vi "Scripting_UpdateViFromTemplate.vi"(0 "ViRef":refnum<vi>, 1 "TemplateVI(Path or Ref)":variant, 5 "error in (no error)":errorcluster) -> (15 "TemplateVersionUsed":string, 19 "error out":errorcluster={"status"=TRUE, "code"=1055, "source"="Property Node in Scripting_ConvertBaseClassToSubClass.vi"})   [LabVIEW 2020]
uses:
  <vilib>/Utility/miscctls.llb/LVRectTypeDef.ctl
  <vilib>/Utility/miscctls.llb/LVPositionTypeDef.ctl
  b5d46679-8400-4ee0-8a03-e36cc4015ed4.vi
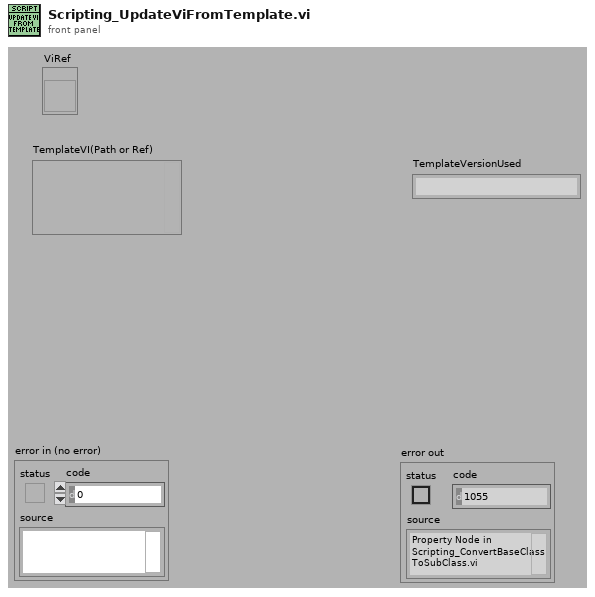
[diagram p1: front panel]
types:
  T1 = typedef "LVRectTypeDef.ctl" = cluster{"Left":i16, "Top":i16, "Right":i16, "Bottom":i16}
  T2 = typedef "LVPositionTypeDef.ctl" = cluster{"Left":i32, "Top":i32}
  T3 = cluster{"ViRef":refnum<vi>, "TemplateRef":refnum<vi>, "ConnectorPaneSettings":cluster{i32, "Wire Rule":enum16{"Invalid Wire Rule", "Required", "Recommended", "Optional", "Dynamic Dispatch"}}[], "ConnectorPaneControlsLabels":string[], "ViClassPath":path, "TemplateViClassPath":path, "ViRootBaseClassPath":path, "TemplateRootBaseClassPath":path, "ClassName":string, "TemplateMemberDataPath":path, "TemplateFile":path, "TemplateVersionUsed":string, "Class":refnum<vi>, "TemplateClassName":string, "permissions":i16, "TemplateClass":refnum<vi>, "Master Bounds Rect":T1, "Visible":bool[], "Controls":refnum<vi>[], "Positions":T2[]}
  T4 = enum32{"invalid lock state", "Not Locked", "Locked (No Password)", "Password-protected"}
  T5 = enum32{"invalid VI type", "Standard VI", "Control VI", "Global VI", "Polymorphic VI", "Configuration VI", "SubSystem", "Facade VI", "Method VI", "Statechart Diagram VI"}
  T6 = enum32{"invalid VI type", "Standard VI", "Control VI", "Global VI", "Polymorphic VI", "Configuration VI", "SubSystem", "Facade VI", "Method VI"}
  T7 = cluster{"Major":u16, "Minor":u16, "Fix":u16, "Build":u16}
  T8 = enum16{"Invalid Wire Rule", "Required", "Recommended", "Optional", "Dynamic Dispatch"}[]
  T9 = cluster{i32, "Wire Rule":enum16{"Invalid Wire Rule", "Required", "Recommended", "Optional", "Dynamic Dispatch"}}
  T10 = cluster{"Position":T2, "Label.Text":string, "Visible":bool, cluster{i32, "Wire Rule":enum16{"Invalid Wire Rule", "Required", "Recommended", "Optional", "Dynamic Dispatch"}}}
  T11 = cluster{"Position":T2, "Label.Text":string, "Visible":bool, cluster{i32, "Wire Rule":enum16{"Invalid Wire Rule", "Required", "Recommended", "Optional", "Dynamic Dispatch"}}}[]
  T12 = cluster{i32, "Wire Rule":enum16{"Invalid Wire Rule", "Required", "Recommended", "Optional", "Dynamic Dispatch"}}[]
  T13 = cluster{"Position":T2, refnum<vi>, "Label.Text":string}
  T14 = cluster{"Position":T2, refnum<vi>, "Label.Text":string}[]
  T15 = enum16{"Invalid Wire Rule", "Required", "Recommended", "Optional", "Dynamic Dispatch"}
  T16 = enum32{"Bad", "Idle", "Run top level", "Running"}
  T17 = typedef "LVPointTypeDef.ctl" = cluster{"Horizontal":i16, "Vertical":i16}
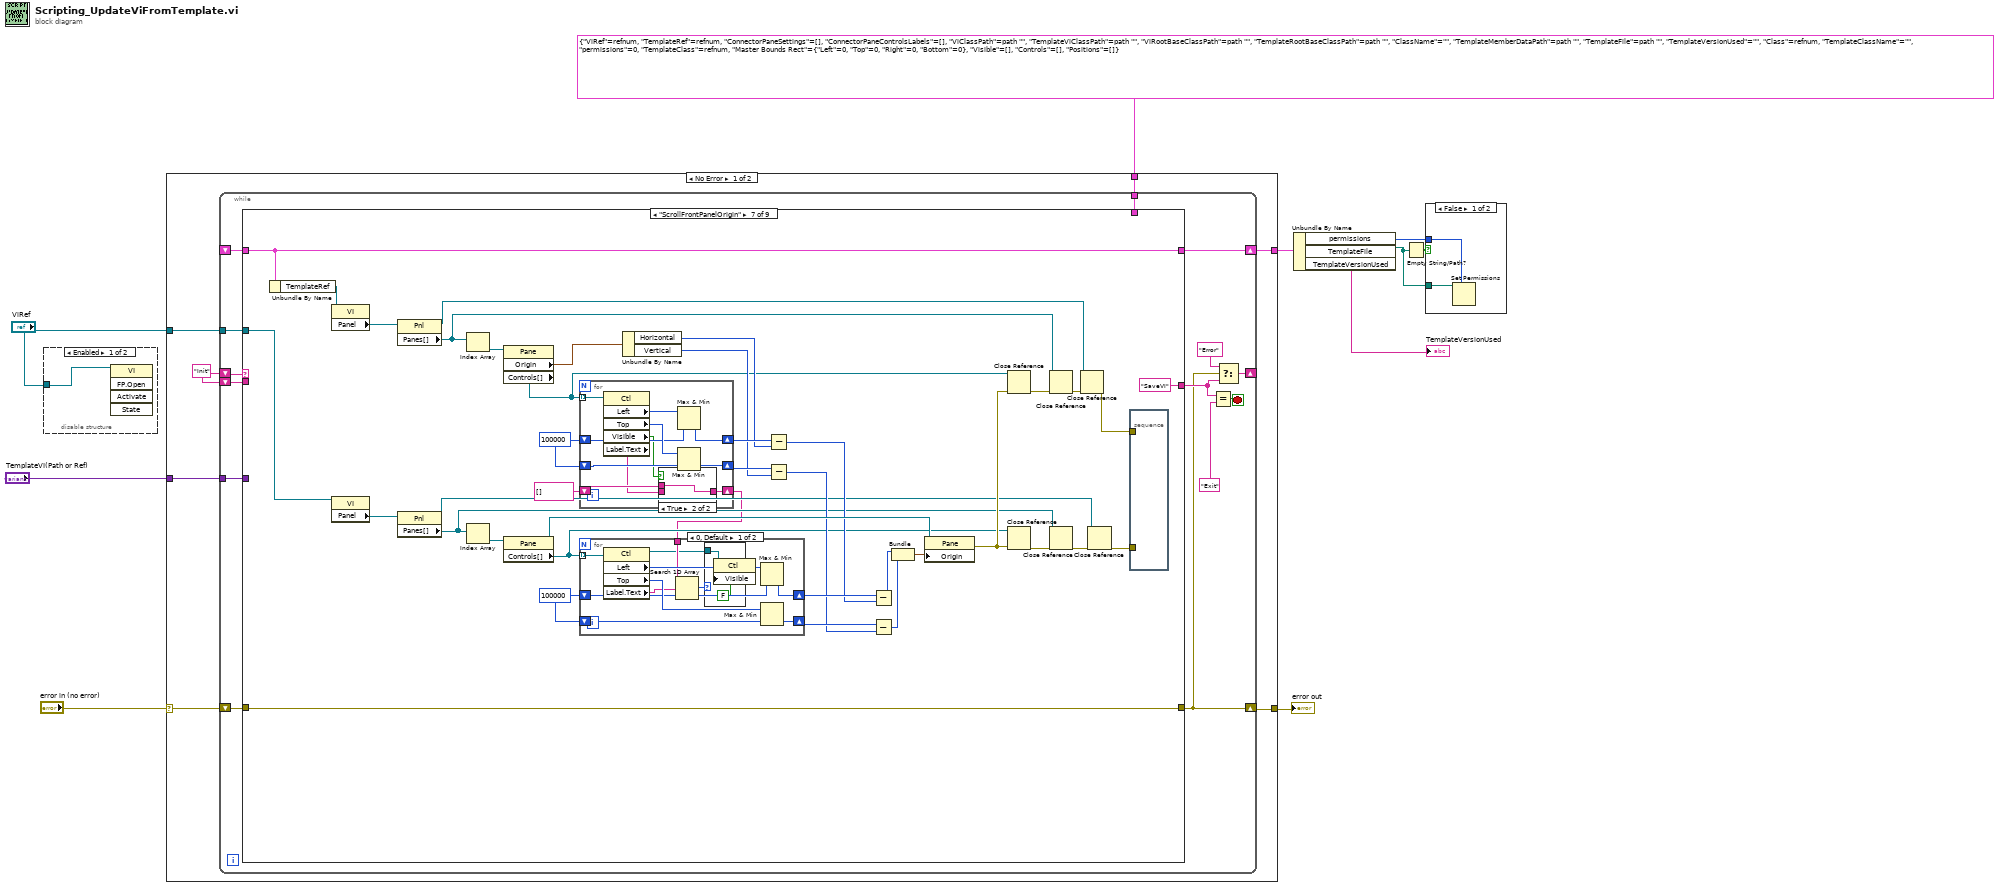
[diagram p0: block diagram]
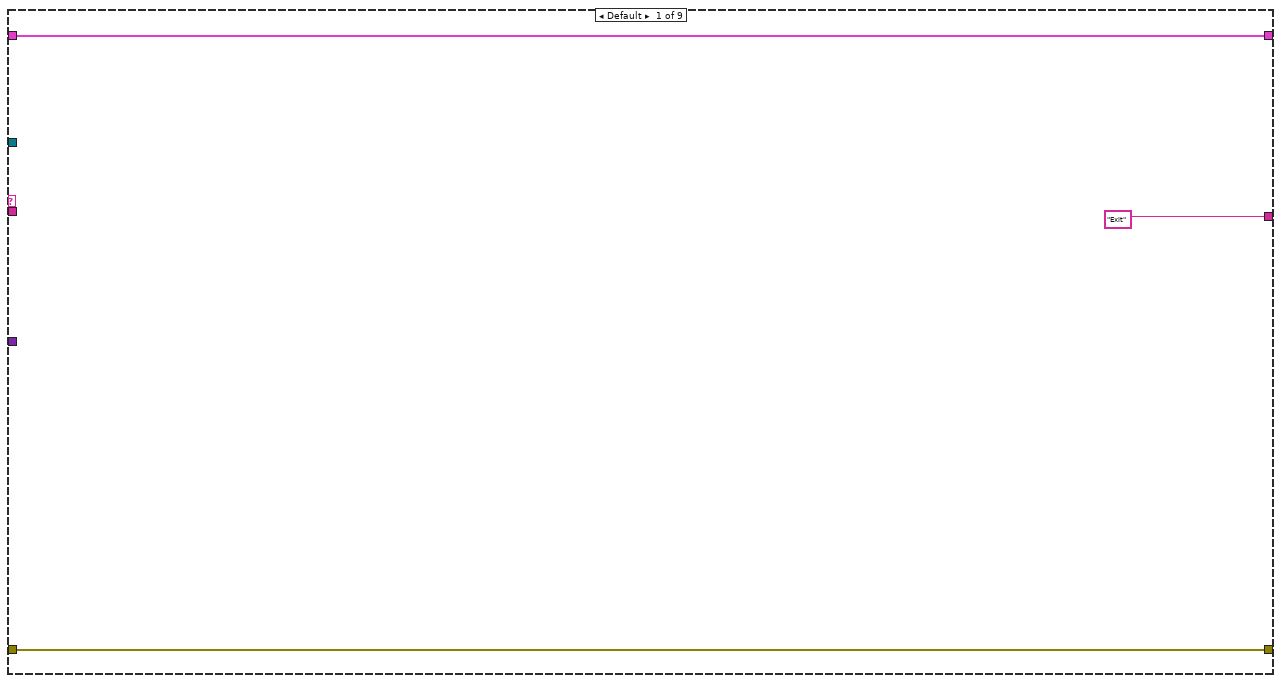
[diagram p4: hidden frame]
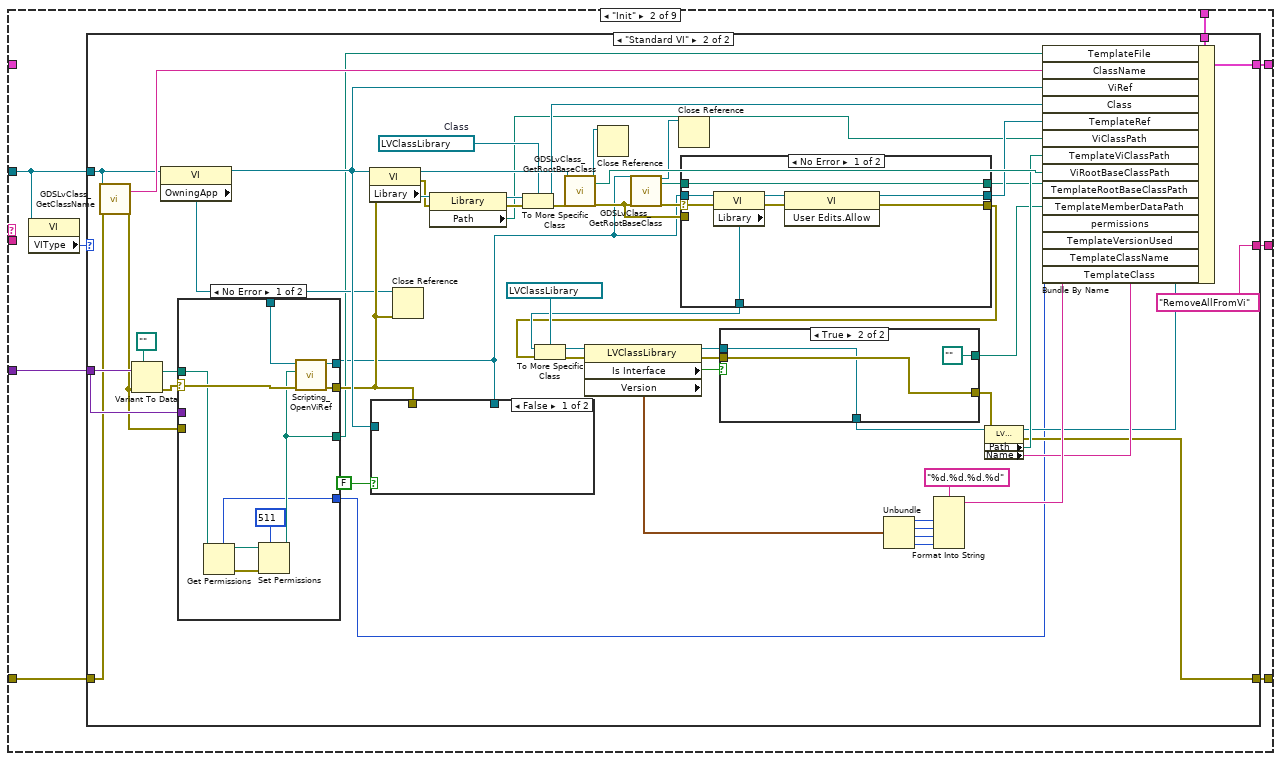
[diagram p5: hidden frame]
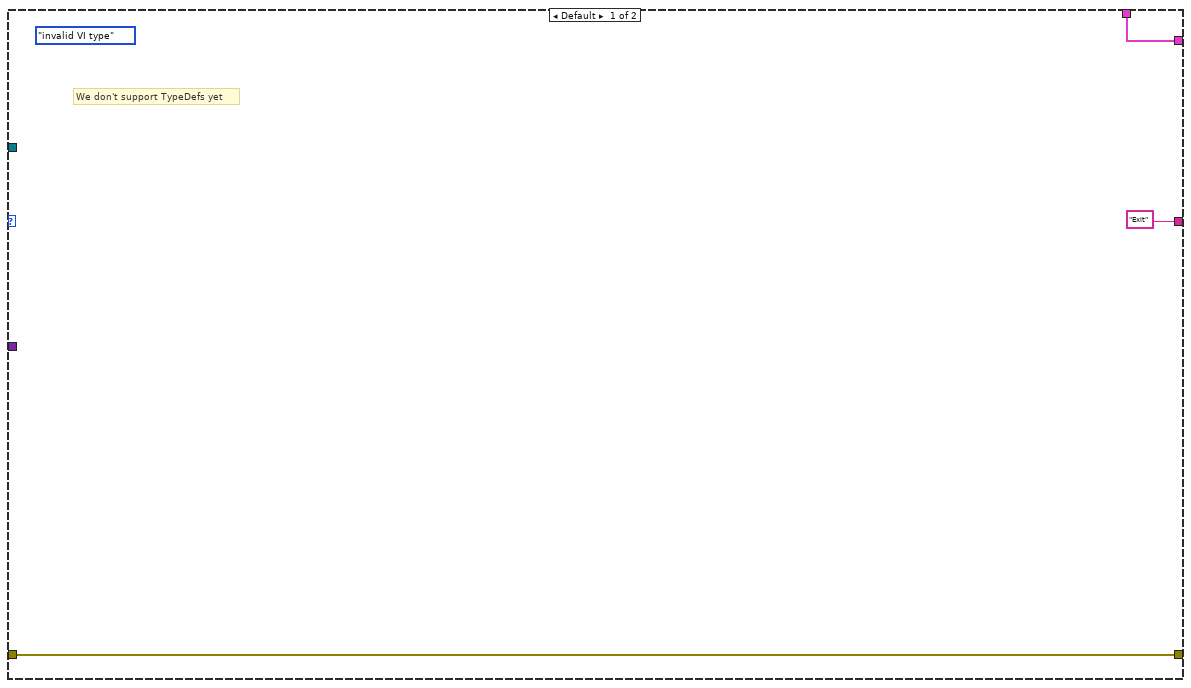
[diagram p6: hidden frame]
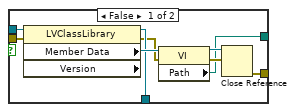
[diagram p7: hidden frame]
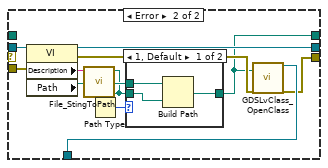
[diagram p8: hidden frame]
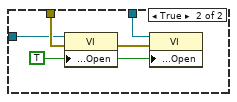
[diagram p10: hidden frame]
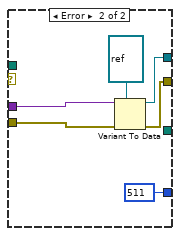
[diagram p11: hidden frame]
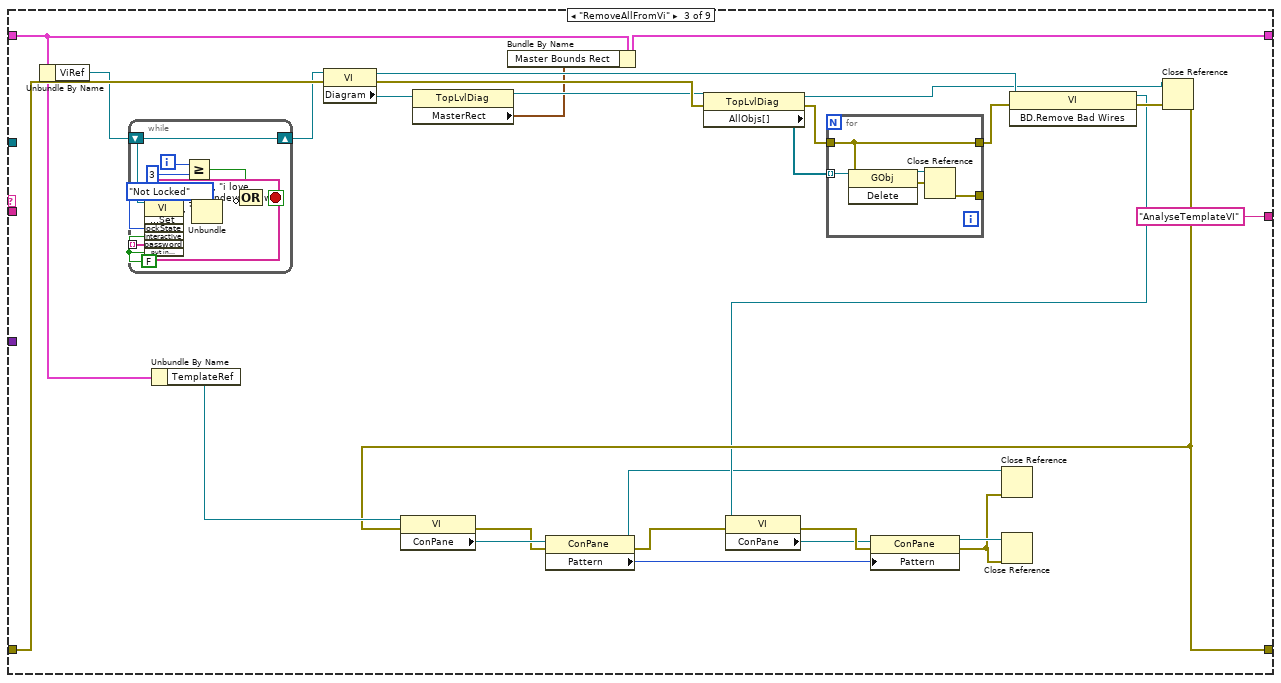
[diagram p12: hidden frame]
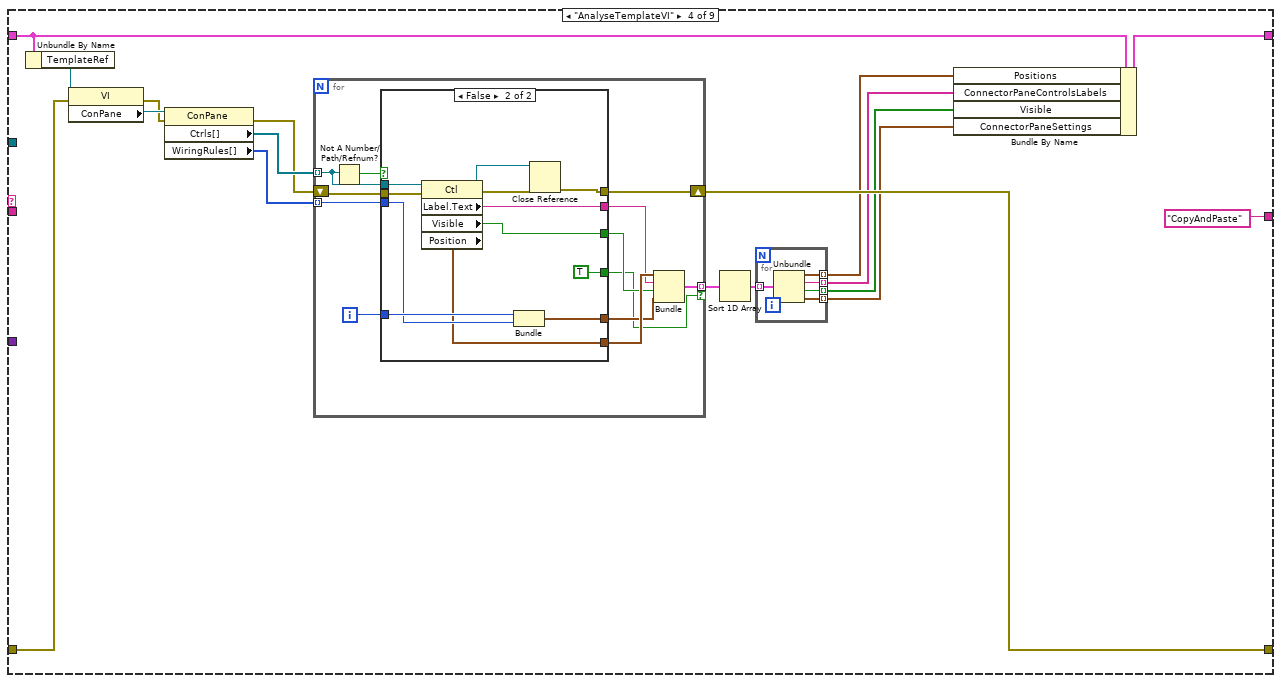
[diagram p13: hidden frame]
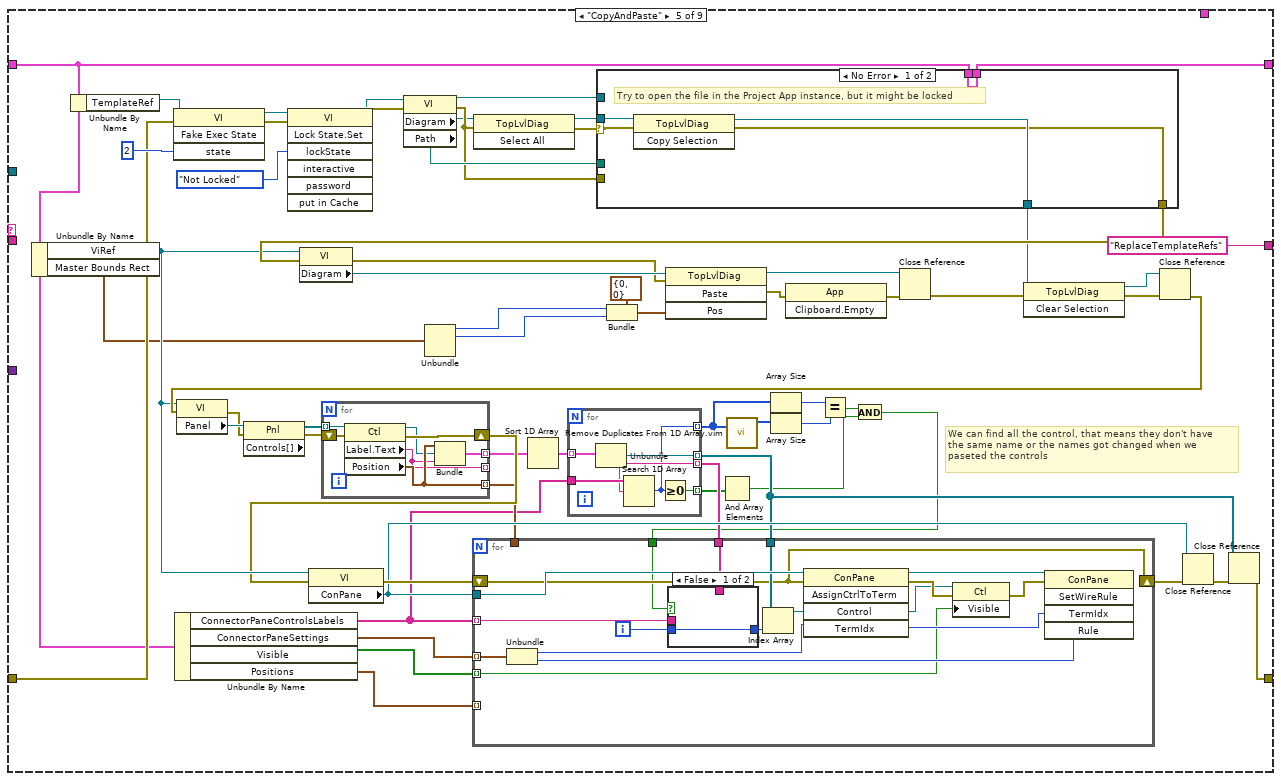
[diagram p15: hidden frame]
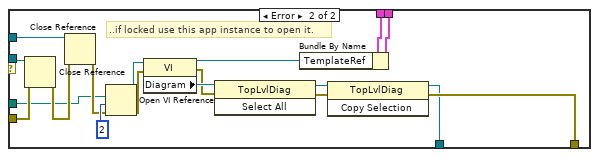
[diagram p16: hidden frame]
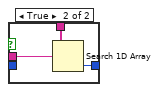
[diagram p17: hidden frame]
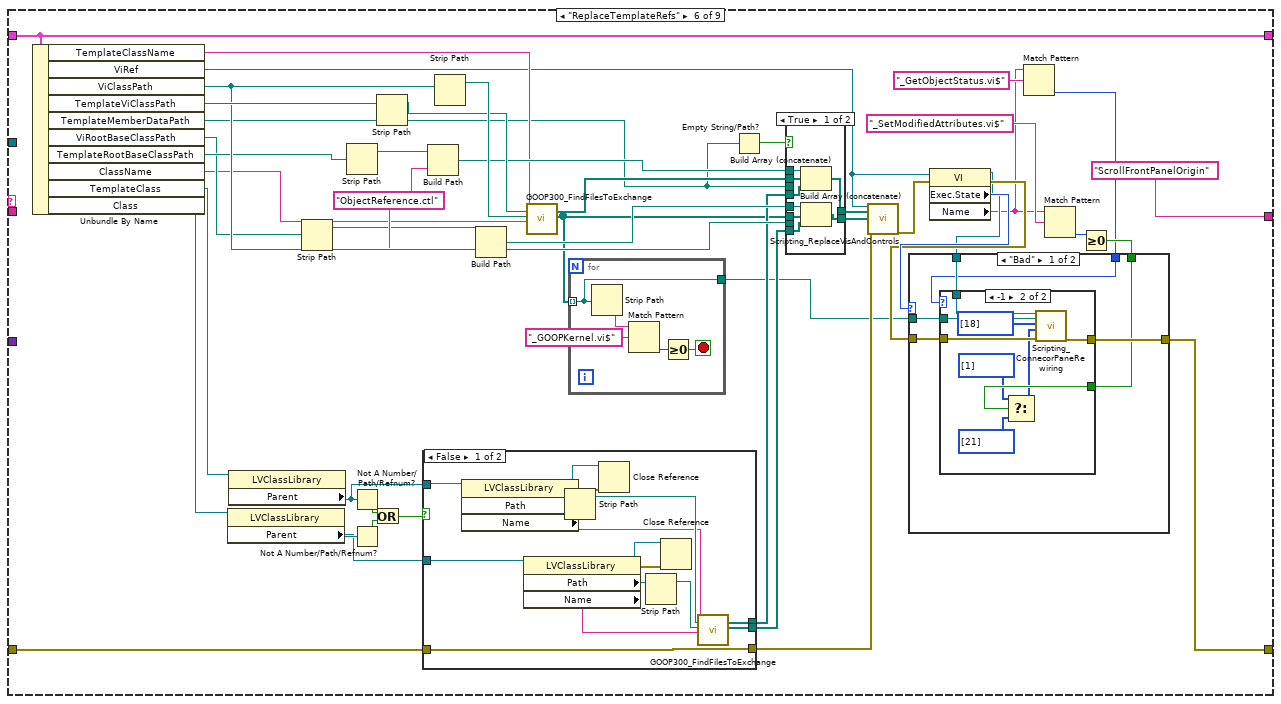
[diagram p18: hidden frame]
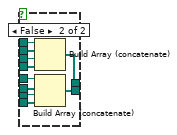
[diagram p19: hidden frame]
diagram:
  n1 = disable-structure shown="Enabled" {
    disable-tunnel: "ViRef" -> [w11 _]
    frame Enabled {
      n2 = invoke class="VI" method="FP.Open"(reference=w11) -> ()  [unwired: 4 in, 5 out]
    }
    frame Disabled {
    }
  }
  n3 = case shown="No Error" "error in (no error)" {
    selector: "error in (no error)" -> [w13 w583]
    tunnel: [w18 w583] -> w10
    tunnel: T3 {"ViRef"=refnum, "TemplateRef"=refnum, "ConnectorPaneSettings"=[], "ConnectorPaneControlsLabels"=[], "ViClassPath"=path "", "TemplateViClassPath"=path "", "ViRootBaseClassPath"=path "", "TemplateRootBaseClassPath"=path "", "ClassName"="", "TemplateMemberDataPath"=path "", "TemplateFile"=path "", "TemplateVersionUsed"="", "Class"=refnum, "TemplateClassName"="", "permissions"=0, "TemplateClass"=refnum, "Master Bounds Rect"={"Left"=0, "Top"=0, "Right"=0, "Bottom"=0}, "Visible"=[], "Controls"=[], "Positions"=[]} -> [w17 _]
    tunnel: "ViRef" -> [w16 _]
    tunnel: "TemplateVI(Path or Ref)" -> [w15 _]
    tunnel: [w12 _] -> w6
    frame No Error {
      w14 = "Init"
      n4 = while {
        shift-right: [w20] -> w18
        shift-left: w13 -> [w22]
        shift-right: [w32] -> _
        shift-left: w14 -> [w27]
        shift-right: [w21] -> w12
        shift-left: _ -> [w26]
        tunnel: w16 -> [w24]
        tunnel: w17 -> [w25]
        tunnel: w15 -> [w23]
        shift-left: w14 -> [w19]
        stop <- w31 stop-if-true
        n5 = case shown="\"ScrollFrontPanelOrigin\"" w27 {
          tunnel: w22 -> [w35 w39 w186 w215 w298 w374 w507 w538 w544]
          tunnel: [w35 w38 w167 w210 w268 w371 w507 w537 w547] -> w20
          tunnel: ["Exit" w43 "AnalyseTemplateVI" "CopyAndPaste" "ReplaceTemplateRefs" "ScrollFrontPanelOrigin" "SaveVI" "CloseReferences" "Exit"] -> w28
          tunnel: [w33 w42 w173 w217 w290 w373 w476 w540 w543] -> w21
          tunnel: w26 -> [w33 _ w171 w218 w284 w373 w476 w540 w543]
          tunnel: w24 -> [_ w37 _ _ _ _ w472 _ w552]
          tunnel: w25 -> [_ w41 _ _ _ _ _ _ _]
          tunnel: w23 -> [_ w40 _ _ _ _ _ _ w554]
          tunnel: w19 -> [_ _ _ _ _ _ _ _ w542]
          frame Default {
          }
          frame "Init" {
            n6 = property class="VI"(reference=w37) -> ("VIType"=w36:T5)  [unwired: 1 in, 2 out]
            n7 = case shown="\"Standard VI\"" w36 {
              tunnel: ["Exit" "RemoveAllFromVi"] -> w43
              tunnel: [w46 w102] -> w42
              tunnel: w41 -> [w46 w101]
              tunnel: w40 -> [_ w97]
              tunnel: w39 -> [w44 w88]
              tunnel: [w44 w64] -> w38
              tunnel: w37 -> [_ w62]
              frame Default {
                (unwired) T6."invalid VI type" ("VIType")
                # "We don't support TypeDefs yet"
              }
              frame "Standard VI" {
                w68 = refnum<vi> refnum  # Class
                n8 = call <resource>:"GDSLvClass_GetClassName.vi"("ViRef/Path,LvClassRef/Path"=w62, "error in (no error)"=w88) -> ("ClassName(without .lvclass)"=w87:string, "error out"=w85:errorcluster)  [unwired: 15 in, 1 out]
                n9 = Variant To Data(error in=w85, type=path "", Variant=w97) -> (data=w98:path, error out=w99:errorcluster)
                n10 = property class="VI"(reference=w62) -> (reference out=w82:refnum<vi>, "OwningApp"=w80:refnum<vi>)  [unwired: 1 in, 1 out]
                n11 = case shown="No Error" w99 {
                  selector: w99 -> [w152 _]
                  tunnel: w98 -> [w145 _]
                  tunnel: [w151 w155] -> w53
                  tunnel: [w150 w154] -> w81
                  tunnel: w85 -> [_ w158]
                  tunnel: w97 -> [_ w157]
                  tunnel: w80 -> [w149 _]
                  tunnel: [w147 _] -> w77
                  tunnel: [w143 i16 511 ("permissions")] -> w60
                  frame No Error {
                    n12 = Get Permissions(11:w145) -> (0:w146:errorcluster, 3:w144:path, 5:w143:i16)  [unwired: 1 in, 2 out]
                    n13 = Set Permissions(7:i16 511 ("permissions"), 8:w146, 11:w144) -> (3:w147:path)  [unwired: 2 in, 1 out]
                    n14 = call <resource>:"Scripting_OpenViRef.vi"("error in"=w152, "ViPath/ViName/Viref"=w147, "AppRef"=w149) -> ("error out"=w150:errorcluster, "vi reference"=w151:refnum<vi>)  [unwired: 6 in, 1 out]
                  }
                  frame Error {
                    n15 = Variant To Data(error in=w158, type=refnum<vi> refnum ("ViRef"), Variant=w157) -> (data=w155:refnum<vi>, error out=w154:errorcluster)
                  }
                }
                n16 = property class="VI"(reference=w82, error in=w81) -> (reference out=w95:refnum<vi>, error out=w84:errorcluster, "Library"=w96:refnum<vi>)
                n17 = case shown="False" FALSE {
                  tunnel: w81 -> [_ w140]
                  tunnel: w53 -> [_ w139]
                  tunnel: w82 -> [_ w138]
                  frame False {
                  }
                  frame True {
                    w141 = TRUE ("Front Panel Window:Open")
                    n18 = property class="VI"(reference=w138, error in=w140, "Front Panel.Open"=w141) -> (error out=w142:errorcluster)  [unwired: 1 out]
                    n19 = property class="VI"(reference=w139, error in=w142, "Front Panel.Open"=w141) -> ()  [unwired: 2 out]
                  }
                }
                n20 = Close Reference(reference=w80, error in (no error)=w81) -> ()  [unwired: 1 out]
                n21 = property class="Library"(reference=w96, error in=w84) -> (reference out=w70:refnum<vi>, error out=w69:errorcluster, "Path"=w59:path)
                n22 = To More Specific Class(target class=w68, reference=w70, error in=w69) -> (specific class reference=w66:refnum<vi>, error out=w67:errorcluster)
                n23 = call <resource>:"GDSLvClass_GetRootBaseClass.vi"("ViRef/Path,LvClassRef/Path"=w95, "error in (no error)"=w67) -> ("RootBaseClassRef"=w94:refnum<vi>, "RootBaseClassPath"=w93:path, "error out"=w57:errorcluster)  [unwired: 11 in, 4 out]
                n24 = Close Reference(reference=w94) -> ()  [unwired: 1 in, 1 out]
                n25 = call <resource>:"GDSLvClass_GetRootBaseClass.vi"("ViRef/Path,LvClassRef/Path"=w53, "error in (no error)"=w57) -> ("RootBaseClassRef"=w61:refnum<vi>, "RootBaseClassPath"=w56:path, "error out"=w58:errorcluster)  [unwired: 11 in, 4 out]
                n26 = Close Reference(reference=w61) -> ()  [unwired: 1 in, 1 out]
                n27 = case shown="No Error" w58 {
                  selector: w58 -> [w117 _]
                  tunnel: [w123 w129] -> w91
                  tunnel: [w122 w133] -> w79
                  tunnel: [w120 w128] -> w78
                  tunnel: w53 -> [w118 w133]
                  tunnel: w57 -> [_ w132]
                  tunnel: w56 -> [w116 _]
                  tunnel: [w116 w124] -> w55
                  frame No Error {
                    n28 = property class="VI"(reference=w118, error in=w117) -> (reference out=w119:refnum<vi>, error out=w121:errorcluster, "Library"=w123:refnum<vi>)
                    n29 = invoke class="VI" method="User Edits.Allow"(reference=w119, error in=w121) -> (reference out=w122:refnum<vi>, error out=w120:errorcluster)  [unwired: 1 in, 1 out]
                  }
                  frame Error {
                    n30 = property class="VI"(reference=w133, error in=w132) -> (error out=w130:errorcluster, "Description"=w131:string, "Path"=w127:path)  [unwired: 1 out]
                    n31 = call <resource>:"File_StingToPath.vi"("Description"=w131) -> ("Path"=w126:path)  [unwired: 10 in]
                    n32 = Path Type(1:w126) -> (0:w125:i16)
                    n33 = case shown="1, Default" w125 {
                      tunnel: w126 -> [w134 w137]
                      tunnel: [w136 w137] -> w124
                      tunnel: w127 -> [w135 _]
                      frame 1, Default {
                        n34 = Build Path(base path=w135, name or relative path=w134) -> (appended path=w136:path)
                      }
                      frame 0 {
                      }
                    }
                    n35 = call <resource>:"GDSLvClass_OpenClass.vi"("ClassToOpen"=w124, "error in (no error)"=w130) -> ("LVClass.Open"=w129:refnum<vi>, "error out"=w128:errorcluster)  [unwired: 16 in]
                  }
                }
                n36 = To More Specific Class(target class=refnum<vi> refnum ("LVClass.Open"), reference=w91, error in=w78) -> (specific class reference=w52:refnum<vi>, error out=w51:errorcluster)
                n37 = property class="LVClassLibrary"(reference=w52, error in=w51) -> (reference out=w50:refnum<vi>, error out=w49:errorcluster, "Is Interface"=w47:bool, "Version"=w48:T7)
                n38 = case shown="True" w47 {
                  tunnel: [w110 w113] -> w90
                  tunnel: [w109 w115] -> w89
                  tunnel: [w106 path "" ("Path")] -> w54
                  tunnel: w50 -> [w105 w113]
                  tunnel: w49 -> [w104 w115]
                  frame False {
                    n39 = property class="LVClassLibrary" props=["Member Data", "Version"](reference=w105, error in=w104) -> (reference out=w110:refnum<vi>, error out=w108:errorcluster, "Member Data"=w111:refnum<vi>)  [unwired: 1 out]
                    n40 = property class="VI"(reference=w111, error in=w108) -> (reference out=w107:refnum<vi>, error out=w112:errorcluster, "Path"=w106:path)
                    n41 = Close Reference(reference=w107, error in (no error)=w112) -> (error out=w109:errorcluster)
                  }
                  frame True {
                  }
                }
                n42 = Unbundle(w48) -> ("Major"=w76:u16, "Minor"=w75:u16, "Fix"=w74:u16, "Build"=w73:u16)
                n43 = Format Into String(format string="%d.%d.%d.%d", w76, w75, w74, w73) -> (resulting string=w71:string)  [unwired: 2 in, 1 out]
                n44 = property class="LVClassLibrary"(reference=w90, error in=w89) -> (reference out=w63:refnum<vi>, error out=w64:errorcluster, "Path"=w86:path, "Name"=w65:string)
                n45 = Bundle By Name(cluster=w101, "TemplateFile"=w77, "ClassName"=w87, "ViRef"=w82, "Class"=w66, "TemplateRef"=w79, "ViClassPath"=w59, "TemplateViClassPath"=w86, "ViRootBaseClassPath"=w93, "TemplateRootBaseClassPath"=w55, "TemplateMemberDataPath"=w54, "permissions"=w60, "TemplateVersionUsed"=w71, "TemplateClassName"=w65, "TemplateClass"=w63) -> (w102:T3)
              }
            }
          }
          frame "RemoveAllFromVi" {
            n46 = Unbundle By Name(w171) -> ("ViRef"=w177:refnum<vi>)
            n47 = while {
              tunnel: string[] ["goop rules", "i love goteborg", "Endevo Knows Goop!", "kiss"] -> [w195] mode=indexing
              shift-right: [w188] -> w176
              shift-left: w177 -> [w188]
              i -> [w192]
              stop <- w193 stop-if-true
              w196 = FALSE ("Interactive")
              n48 = invoke class="VI" method="Lock State.Set"(reference=w188, "lockState"=T4."Not Locked" ("Lock State"), "interactive"=w196, "password"=w195, "put in Cache"=w196) -> (error out=w194:errorcluster)  [unwired: 2 in, 6 out]
              n49 = Greater Or Equal?(x=w192, y=3) -> (x >= y?=w191:bool)
              n50 = Unbundle(w194) -> ("status"=w189:bool)  [unwired: 2 out]
              n51 = Compound Arithmetic op=OR(w191, invert w189) -> (w193:bool)
            }
            n52 = Unbundle By Name(w171) -> ("TemplateRef"=w168:refnum<vi>)
            n53 = property class="VI"(reference=w176, error in=w186) -> (reference out=w184:refnum<vi>, error out=w181:errorcluster, "Diagram"=w175:refnum<vi>)
            n54 = property class="TopLvlDiag"(reference=w175) -> (reference out=w174:refnum<vi>, "MasterRect"=w172:T1)  [unwired: 1 in, 1 out]
            n55 = Bundle By Name(cluster=w171, "Master Bounds Rect"=w172) -> (w173:T3)
            n56 = property class="TopLvlDiag"(reference=w174, error in=w181) -> (reference out=w179:refnum<vi>, error out=w183:errorcluster, "AllObjs[]"=w182:refnum<vi>[])
            n57 = for {
              tunnel: w183 -> [w200]
              tunnel: w182 -> [w201] mode=indexing
              tunnel: [w200] -> w180
              tunnel: [w198] -> _
              n58 = invoke class="GObj" method="Delete"(reference=w201, error in=w200) -> (reference out=w202:refnum<vi>, error out=w199:errorcluster)  [unwired: 1 in, 1 out]
              n59 = Close Reference(reference=w202, error in (no error)=w199) -> (error out=w198:errorcluster)
            }
            n60 = invoke class="VI" method="BD.Remove Bad Wires"(reference=w184, error in=w180) -> (reference out=w163:refnum<vi>, error out=w185:errorcluster)  [unwired: 1 in, 1 out]
            n61 = Close Reference(reference=w179, error in (no error)=w185) -> (error out=w167:errorcluster)
            n62 = property class="VI"(reference=w168, error in=w167) -> (error out=w169:errorcluster, "ConPane"=w170:refnum<vi>)  [unwired: 1 out]
            n63 = property class="ConPane"(reference=w170, error in=w169) -> (reference out=w161:refnum<vi>, error out=w164:errorcluster, "Pattern"=w162:u32)
            n64 = property class="VI"(reference=w163, error in=w164) -> (error out=w166:errorcluster, "ConPane"=w165:refnum<vi>)  [unwired: 1 out]
            n65 = property class="ConPane"(reference=w165, error in=w166, "Pattern"=w162) -> (reference out=w160:refnum<vi>, error out=w159:errorcluster)
            n66 = Close Reference(reference=w161, error in (no error)=w159) -> ()  [unwired: 1 out]
            n67 = Close Reference(reference=w160, error in (no error)=w159) -> ()  [unwired: 1 out]
          }
          frame "AnalyseTemplateVI" {
            n68 = Unbundle By Name(w218) -> ("TemplateRef"=w216:refnum<vi>)
            n69 = property class="VI"(reference=w216, error in=w215) -> (error out=w209:errorcluster, "ConPane"=w214:refnum<vi>)  [unwired: 1 out]
            n70 = property class="ConPane"(reference=w214, error in=w209) -> (error out=w211:errorcluster, "Ctrls[]"=w213:refnum<vi>[], "WiringRules[]"=w212:T8)  [unwired: 1 out]
            n71 = for {
              tunnel: w213 -> [w234] mode=indexing
              tunnel: w212 -> [w232] mode=indexing
              shift-right: [w231] -> w210
              shift-left: w211 -> [w235]
              tunnel: [w226] -> w208 mode=indexing if=w225
              i -> [w233]
              n72 = Not A Number/Path/Refnum?(number/path/refnum=w234) -> (NaN/Path/Refnum?=w236:bool)
              n73 = case shown="False" w236 {
                tunnel: w235 -> [w237 w249]
                tunnel: w234 -> [_ w248]
                tunnel: w233 -> [_ w247]
                tunnel: w232 -> [_ w246]
                tunnel: [w237 w243] -> w231
                tunnel: [_ w242] -> w229
                tunnel: [_ w241] -> w228
                tunnel: [_ w240] -> w227
                tunnel: [_ w239] -> w230
                tunnel: [_ TRUE] -> w225
                frame True {
                }
                frame False {
                  n74 = property class="Ctl"(reference=w248, error in=w249) -> (reference out=w244:refnum<vi>, error out=w245:errorcluster, "Label.Text"=w242:string, "Visible"=w241:bool, "Position"=w239:T2)
                  n75 = Bundle(w247, "Wire Rule"=w246) -> (w240:T9)  [unwired: 1 in]
                  n76 = Close Reference(reference=w244, error in (no error)=w245) -> (error out=w243:errorcluster)
                }
              }
              n77 = Bundle("Position"=w230, "Label.Text"=w229, "Visible"=w228, w227) -> (w226:T10)  [unwired: 1 in]
            }
            n78 = Sort 1D Array(array=w208) -> (sorted array=w207:T11)
            n79 = for {
              tunnel: w207 -> [w224] mode=indexing
              tunnel: [w223] -> w206 mode=indexing
              tunnel: [w222] -> w205 mode=indexing
              tunnel: [w221] -> w204 mode=indexing
              tunnel: [w220] -> w203 mode=indexing
              n80 = Unbundle(w224) -> ("Position"=w223:T2, "Label.Text"=w222:string, "Visible"=w221:bool, w220:T9)
            }
            n81 = Bundle By Name(cluster=w218, "Positions"=w206, "ConnectorPaneControlsLabels"=w205, "Visible"=w204, "ConnectorPaneSettings"=w203) -> (w217:T3)
          }
          frame "CopyAndPaste" {
            # "We can find all the control, that means they don't have\nthe same name or the names got changed when we\npaseted the controls"
            n82 = Unbundle By Name(w284) -> ("ViRef"=w282:refnum<vi>, "Master Bounds Rect"=w276:T1)
            n83 = Unbundle By Name(w284) -> ("TemplateRef"=w299:refnum<vi>)
            n84 = invoke class="VI" method="Fake Exec State"(reference=w299, error in=w298, "state"=2 ("State")) -> (reference out=w294:refnum<vi>, error out=w297:errorcluster)  [unwired: 1 in, 2 out]
            n85 = Unbundle By Name(w284) -> ("ConnectorPaneControlsLabels"=w258:string[], "ConnectorPaneSettings"=w303:T12, "Visible"=w267:bool[], "Positions"=w266:T2[])
            n86 = invoke class="VI" method="Lock State.Set"(reference=w294, "lockState"=T4."Not Locked" ("Lock State")) -> (reference out=w295:refnum<vi>)  [unwired: 5 in, 6 out]
            n87 = property class="VI"(reference=w295, error in=w297) -> (reference out=w283:refnum<vi>, error out=w291:errorcluster, "Diagram"=w281:refnum<vi>, "Path"=w292:path)
            n88 = Unbundle(w276) -> ("Left"=w275:i16, "Top"=w274:i16)  [unwired: 2 out]
            n89 = invoke class="TopLvlDiag" method="Select All"(reference=w281, error in=w291) -> (reference out=w308:refnum<vi>, error out=w293:errorcluster)  [unwired: 1 in, 1 out]
            n90 = case shown="No Error" w293 {
              selector: w293 -> [w319 _]
              tunnel: w308 -> [w320 w332]
              tunnel: [w316 w327] -> w285
              tunnel: w292 -> [_ w323]
              tunnel: w291 -> [_ w331]
              tunnel: w284 -> [w318 w336]
              tunnel: [w318 w335] -> w290
              tunnel: [w317 w326] -> w272
              tunnel: w283 -> [_ w333]
              frame No Error {
                # "Try to open the file in the Project App instance, but it might be locked"
                n91 = invoke class="TopLvlDiag" method="Copy Selection"(reference=w320, error in=w319) -> (reference out=w317:refnum<vi>, error out=w316:errorcluster)  [unwired: 1 in, 1 out]
              }
              frame Error {
                # "..if locked use this app instance to open it."
                n92 = Close Reference(reference=w332, error in (no error)=w331) -> (error out=w330:errorcluster)
                n93 = Close Reference(reference=w333, error in (no error)=w330) -> (error out=w324:errorcluster)
                n94 = Open VI Reference(vi path=w323, options=2, error in (no error)=w324) -> (vi reference=w321:refnum<vi>, error out=w322:errorcluster)  [unwired: 3 in]
                n95 = property class="VI"(reference=w321, error in=w322) -> (reference out=w334:refnum<vi>, error out=w337:errorcluster, "Diagram"=w338:refnum<vi>)
                n96 = invoke class="TopLvlDiag" method="Select All"(reference=w338, error in=w337) -> (reference out=w329:refnum<vi>, error out=w328:errorcluster)  [unwired: 1 in, 1 out]
                n97 = Bundle By Name(cluster=w336, "TemplateRef"=w334) -> (w335:T3)
                n98 = invoke class="TopLvlDiag" method="Copy Selection"(reference=w329, error in=w328) -> (reference out=w326:refnum<vi>, error out=w327:errorcluster)  [unwired: 1 in, 1 out]
              }
            }
            n99 = property class="VI"(reference=w282, error in=w285) -> (error out=w277:errorcluster, "Diagram"=w278:refnum<vi>)  [unwired: 1 out]
            n100 = Bundle(cluster=T2 {"Left"=0, "Top"=0} ("Position"), "Left"=w275, "Top"=w274) -> (w279:T2)
            n101 = invoke class="TopLvlDiag" method="Paste"(reference=w278, error in=w277, "Pos"=w279) -> (reference out=w288:refnum<vi>, error out=w287:errorcluster)  [unwired: 1 in, 2 out]
            n102 = invoke class="App" method="Clipboard.Empty"(error in=w287) -> (error out=w289:errorcluster)  [unwired: 2 in, 2 out]
            n103 = Close Reference(reference=w288, error in (no error)=w289) -> (error out=w271:errorcluster)
            n104 = invoke class="TopLvlDiag" method="Clear Selection"(reference=w272, error in=w271) -> (reference out=w273:refnum<vi>, error out=w270:errorcluster)  [unwired: 1 in, 1 out]
            n105 = Close Reference(reference=w273, error in (no error)=w270) -> (error out=w286:errorcluster)
            n106 = property class="VI"(reference=w282, error in=w286) -> (error out=w305:errorcluster, "Panel"=w306:refnum<vi>)  [unwired: 1 out]
            n107 = property class="Pnl"(reference=w306, error in=w305) -> (error out=w304:errorcluster, "Controls[]"=w261:refnum<vi>[])  [unwired: 1 out]
            n108 = for {
              tunnel: w261 -> [w343] mode=indexing
              shift-right: [w344] -> w265
              shift-left: w304 -> [w345]
              tunnel: [w340] -> _ mode=indexing
              tunnel: [w342] -> w264 mode=indexing
              tunnel: [w339] -> w263 mode=indexing
              n109 = property class="Ctl"(reference=w343, error in=w345) -> (reference out=w341:refnum<vi>, error out=w344:errorcluster, "Label.Text"=w340:string, "Position"=w342:T2)
              n110 = Bundle("Position"=w342, w341, "Label.Text"=w340) -> (w339:T13)  [unwired: 1 in]
            }
            n111 = property class="VI"(reference=w282, error in=w265) -> (error out=w307:errorcluster, "ConPane"=w301:refnum<vi>)  [unwired: 1 out]
            n112 = Sort 1D Array(array=w263) -> (sorted array=w262:T14)
            n113 = for {
              tunnel: w262 -> [w315] mode=indexing
              tunnel: [w314] -> w260 mode=indexing
              tunnel: [w312] -> w259 mode=indexing
              tunnel: w258 -> [w313]
              tunnel: [w311] -> w257 mode=indexing
              tunnel: [w310] -> w255 mode=indexing
              n114 = Unbundle(w315) -> (w314:refnum<vi>, "Label.Text"=w312:string)  [unwired: 1 out]
              n115 = Search 1D Array(1D array=w313, element=w312) -> (index of element=w310:i32)  [unwired: 1 in]
              n116 = Greater Or Equal To 0?(x=w310) -> (x >= 0?=w311:bool)
            }
            n117 = And Array Elements(Boolean array=w257) -> (logical AND=w251:bool)
            n118 = call "Remove Duplicates From 1D Array.vim"("array"=w255) -> ("array with duplicates removed"=w256:i32[])  [unwired: 10 in]
            n119 = Array Size(array=w255) -> (size(s)=w254:i32)
            n120 = Array Size(array=w256) -> (size(s)=w253:i32)
            n121 = Equal?(x=w254, y=w253) -> (x = y?=w252:bool)
            n122 = And(x=w252, y=w251) -> (x .and. y?=w250:bool)
            n123 = for {
              shift-right: [w348] -> w302
              shift-left: w307 -> [w348]
              tunnel: w301 -> [w360]
              tunnel: w258 -> [w359] mode=indexing
              tunnel: w259 -> [w358]
              tunnel: w260 -> [w357]
              tunnel: w303 -> [w355] mode=indexing
              tunnel: w267 -> [w349] mode=indexing
              tunnel: w266 -> [_] mode=indexing
              tunnel: w264 -> [_]
              tunnel: w250 -> [w347]
              i -> [w346]
              n124 = Unbundle(w355) -> (w354:i32, "Wire Rule"=w353:T15)
              n125 = case shown="False" w347 {
                tunnel: [w362 w365] -> w361
                tunnel: w359 -> [_ w364]
                tunnel: w358 -> [_ w363]
                tunnel: w346 -> [w362 _]
                frame False {
                }
                frame True {
                  n126 = Search 1D Array(1D array=w363, element=w364) -> (index of element=w365:i32)  [unwired: 1 in]
                }
              }
              n127 = Index Array(array=w357, index=w361) -> (element=w350:refnum<vi>)
              n128 = invoke class="ConPane" method="AssignCtrlToTerm"(reference=w360, error in=w348, "Control"=w350, "TermIdx"=w354) -> (reference out=w356:refnum<vi>, error out=w351:errorcluster)  [unwired: 1 in, 3 out]
              n129 = property class="Ctl"(reference=w350, error in=w351, "Visible"=w349) -> (error out=w352:errorcluster)  [unwired: 1 out]
              n130 = invoke class="ConPane" method="SetWireRule"(reference=w356, error in=w352, "TermIdx"=w354, "Rule"=w353) -> ()  [unwired: 1 in, 5 out]
            }
            n131 = Close Reference(reference=w301, error in (no error)=w302) -> (error out=w269:errorcluster)
            n132 = Close Reference(reference=w260, error in (no error)=w269) -> (error out=w268:errorcluster)
          }
          frame "ReplaceTemplateRefs" {
            w402 = "ObjectReference.ctl" ("name or relative path")
            n133 = Unbundle By Name(w373) -> ("TemplateClassName"=w397:string, "ViRef"=w384:refnum<vi>, "ViClassPath"=w405:path, "TemplateViClassPath"=w406:path, "TemplateMemberDataPath"=w367:path, "ViRootBaseClassPath"=w399:path, "TemplateRootBaseClassPath"=w404:path, "ClassName"=w396:string, "TemplateClass"=w386:refnum<vi>, "Class"=w385:refnum<vi>)
            n134 = property class="LVClassLibrary"(reference=w385) -> (reference out=w395:refnum<vi>, "Parent"=w390:refnum<vi>)  [unwired: 1 in, 1 out]
            n135 = property class="LVClassLibrary"(reference=w386) -> ("Parent"=w391:refnum<vi>)  [unwired: 1 in, 2 out]
            n136 = Strip Path(path=w399) -> (stripped path=w398:path)  [unwired: 1 out]
            n137 = Strip Path(path=w404) -> (stripped path=w403:path)  [unwired: 1 out]
            n138 = Not A Number/Path/Refnum?(number/path/refnum=w391) -> (NaN/Path/Refnum?=w394:bool)
            n139 = Not A Number/Path/Refnum?(number/path/refnum=w395) -> (NaN/Path/Refnum?=w393:bool)
            n140 = Or(x=w394, y=w393) -> (x .or. y?=w392:bool)
            n141 = Strip Path(path=w406) -> (stripped path=w407:path)  [unwired: 1 out]
            n142 = case shown="False" w392 {
              tunnel: w391 -> [w454 w469]
              tunnel: w390 -> [w466 w468]
              tunnel: [w460 _] -> w389
              tunnel: [w459 _] -> w388
              tunnel: w374 -> [w458 w467]
              tunnel: [w458 w467] -> w387
              frame False {
                n143 = property class="LVClassLibrary"(reference=w454) -> (reference out=w456:refnum<vi>, error out=w455:errorcluster, "Path"=w457:path, "Name"=w452:string)  [unwired: 1 in]
                n144 = property class="LVClassLibrary"(reference=w466) -> (reference out=w464:refnum<vi>, error out=w465:errorcluster, "Path"=w463:path, "Name"=w461:string)  [unwired: 1 in]
                n145 = Strip Path(path=w457) -> (stripped path=w453:path)  [unwired: 1 out]
                n146 = Close Reference(reference=w456, error in (no error)=w455) -> ()  [unwired: 1 out]
                n147 = Strip Path(path=w463) -> (stripped path=w462:path)  [unwired: 1 out]
                n148 = Close Reference(reference=w464, error in (no error)=w465) -> ()  [unwired: 1 out]
                n149 = call <resource>:"GOOP300_FindFilesToExchange.vi"("OldClassName(Prefix or suffix for some VIs)"=w452, "OldFolderPath"=w453, "NewFolderPath"=w462, "NewClassName(Prefix or suffix for some VIs)"=w461) -> ("OldFiles"=w460:path[], "NewFileArray"=w459:path[])  [unwired: 2 in, 12 out]
              }
              frame True {
                n150 = Close Reference(reference=w468) -> ()  [unwired: 1 in, 1 out]
                n151 = Close Reference(reference=w469) -> ()  [unwired: 1 in, 1 out]
              }
            }
            n152 = Build Path(base path=w403, name or relative path=w402) -> (appended path=w401:path)
            n153 = Strip Path(path=w405) -> (stripped path=w408:path)  [unwired: 1 out]
            n154 = Build Path(base path=w398, name or relative path=w402) -> (appended path=w400:path)
            n155 = call <resource>:"GOOP300_FindFilesToExchange.vi"("OldClassName(Prefix or suffix for some VIs)"=w397, "OldFolderPath"=w407, "NewFolderPath"=w408, "NewClassName(Prefix or suffix for some VIs)"=w396) -> ("OldFiles"=w411:path[], "NewFileArray"=w380:path[])  [unwired: 2 in, 12 out]
            n156 = for {
              tunnel: w380 -> [w430] mode=indexing
              tunnel: [w430] -> w379
              stop <- w431 stop-if-true
              n157 = Strip Path(path=w430) -> (name=w434:string)  [unwired: 1 out]
              n158 = Match Pattern(string=w434, regular expression="_GOOPKernel.vi$") -> (offset past match=w432:i32)  [unwired: 1 in, 3 out]
              n159 = Greater Or Equal To 0?(x=w432) -> (x >= 0?=w431:bool)
            }
            n160 = Empty String/Path?(string/path=w367) -> (empty?=w366:bool)
            n161 = case shown="True" w366 {
              tunnel: w411 -> [w419 w429]
              tunnel: [w418 w428] -> w410
              tunnel: [w417 w427] -> w409
              tunnel: w405 -> [_ w426]
              tunnel: w401 -> [w416 w425]
              tunnel: w400 -> [w415 w424]
              tunnel: w389 -> [w414 w423]
              tunnel: w388 -> [w413 w422]
              tunnel: w380 -> [w412 w421]
              tunnel: w367 -> [_ w420]
              frame True {
                n162 = Build Array (concatenate)(w416, w419, w414) -> (w418:path[])
                n163 = Build Array (concatenate)(w415, w412, w413) -> (w417:path[])
              }
              frame False {
                n164 = Build Array (concatenate)(w425, w429, w420, w423) -> (w428:path[])
                n165 = Build Array (concatenate)(w424, w421, w426, w422) -> (w427:path[])
              }
            }
            n166 = call <resource>:"Scripting_ReplaceVisAndControls.vi"("ViRef"=w384, "OldVIsAndControls"=w410, "NewVIsAndControls"=w409, "error in (no error)"=w387) -> ("error out"=w383:errorcluster)  [unwired: 15 out]
            n167 = property class="VI"(reference=w384, error in=w383) -> (reference out=w378:refnum<vi>, error out=w381:errorcluster, "Exec.State"=w382:T16, "Name"=w369:string)
            n168 = Match Pattern(string=w369, regular expression="_GetObjectStatus.vi$") -> (offset past match=w368:i32)  [unwired: 1 in, 3 out]
            n169 = Match Pattern(string=w369, regular expression="_SetModifiedAttributes.vi$") -> (offset past match=w376:i32)  [unwired: 1 in, 3 out]
            n170 = Greater Or Equal To 0?(x=w376) -> (x >= 0?=w375:bool)
            n171 = case shown="\"Bad\"" w382 {
              tunnel: w381 -> [w440 w451]
              tunnel: w379 -> [w439 _]
              tunnel: w378 -> [w438 _]
              tunnel: [w437 w451] -> w371
              tunnel: w375 -> [w436 _]
              tunnel: w368 -> [w435 _]
              frame "Bad" {
                n172 = case shown="-1" w435 {
                  tunnel: w440 -> [w441 w450]
                  tunnel: w439 -> [_ w449]
                  tunnel: w438 -> [_ w448]
                  tunnel: [w441 w446] -> w437
                  tunnel: w436 -> [_ w445]
                  frame 0, Default {
                  }
                  frame -1 {
                    n173 = Select(t=u32[] [1] ("OldConnectorPaneIndex"), s=w445, f=u32[] [21] ("OldConnectorPaneIndex")) -> (s? t:f=w443:u32[])
                    n174 = call <resource>:"Scripting_ConnecorPaneRewiring.vi"("ViRef"=w448, "SubViThatHasChangedConnectorPane"=w449, "OldConnectorPaneIndex"=u32[] [18], "NewConnectorPaneIndex"=w443, "error in (no error)"=w450) -> ("error out"=w446:errorcluster)  [unwired: 14 in]
                  }
                }
              }
              frame "Idle", Default {
              }
            }
          }
          frame "ScrollFrontPanelOrigin" {
            w496 = 100000
            w504 = 100000
            n175 = Unbundle By Name(w476) -> ("TemplateRef"=w475:refnum<vi>)
            n176 = property class="VI"(reference=w475) -> ("Panel"=w506:refnum<vi>)  [unwired: 1 in, 2 out]
            n177 = property class="VI"(reference=w472) -> ("Panel"=w494:refnum<vi>)  [unwired: 1 in, 2 out]
            n178 = property class="Pnl"(reference=w506) -> (reference out=w477:refnum<vi>, "Panes[]"=w485:refnum<vi>[])  [unwired: 1 in, 1 out]
            n179 = property class="Pnl"(reference=w494) -> (reference out=w479:refnum<vi>, "Panes[]"=w480:refnum<vi>[])  [unwired: 1 in, 1 out]
            n180 = Index Array(array=w485) -> (element=w505:refnum<vi>)  [unwired: 1 in]
            n181 = Index Array(array=w480) -> (element=w495:refnum<vi>)  [unwired: 1 in]
            n182 = property class="Pane"(reference=w505) -> ("Origin"=w503:T17, "Controls[]"=w487:refnum<vi>[])  [unwired: 1 in, 2 out]
            n183 = property class="Pane"(reference=w495) -> (reference out=w493:refnum<vi>, "Controls[]"=w481:refnum<vi>[])  [unwired: 1 in, 1 out]
            n184 = for {
              tunnel: w487 -> [w532] mode=indexing
              shift-right: [w528] -> w502
              shift-left: w504 -> [w529]
              shift-right: [w526] -> w500
              shift-left: w504 -> [w527]
              shift-right: [w524] -> w470
              shift-left: string[] [] -> [w523]
              n185 = property class="Ctl"(reference=w532) -> ("Left"=w531:i32, "Top"=w530:i32, "Visible"=w525:bool, "Label.Text"=w522:string)  [unwired: 1 in, 2 out]
              n186 = case shown="True" w525 {
                tunnel: [w535 w536] -> w524
                tunnel: w523 -> [w534 w536]
                tunnel: w522 -> [w533 _]
                frame False {
                  n187 = Build Array (concatenate)(w534, w533) -> (w535:string[])
                }
                frame True {
                }
              }
              n188 = Max & Min(x=w531, y=w529) -> (min(x,y)=w528:i32)  [unwired: 1 out]
              n189 = Max & Min(x=w530, y=w527) -> (min(x,y)=w526:i32)  [unwired: 1 out]
            }
            n190 = for {
              tunnel: w481 -> [w519] mode=indexing
              shift-right: [w515] -> w497
              shift-left: w496 -> [w516]
              shift-right: [w513] -> w498
              shift-left: w496 -> [w514]
              tunnel: w470 -> [w511]
              n191 = property class="Ctl"(reference=w519) -> (reference out=w509:refnum<vi>, "Left"=w518:i32, "Top"=w517:i32, "Label.Text"=w512:string)  [unwired: 1 in, 1 out]
              n192 = Search 1D Array(1D array=w511, element=w512) -> (index of element=w510:i32)  [unwired: 1 in]
              n193 = case shown="0, Default" w510 {
                tunnel: w509 -> [w521 _]
                frame 0, Default {
                  n194 = property class="Ctl"(reference=w521, "Visible"=FALSE) -> ()  [unwired: 1 in, 2 out]
                }
                frame -1 {
                }
              }
              n195 = Max & Min(x=w518, y=w516) -> (min(x,y)=w515:i32)  [unwired: 1 out]
              n196 = Max & Min(x=w517, y=w514) -> (min(x,y)=w513:i32)  [unwired: 1 out]
            }
            n197 = Unbundle By Name(w503) -> ("Horizontal"=w501:i16, "Vertical"=w499:i16)
            n198 = Subtract(x=w502, y=w501) -> (x-y=w492:i32)
            n199 = Subtract(x=w500, y=w499) -> (x-y=w491:i32)
            n200 = Subtract(x=w497, y=w492) -> (x-y=w490:i32)
            n201 = Subtract(x=w498, y=w491) -> (x-y=w489:i32)
            n202 = Bundle(w490, w489) -> (w488:cluster{i32, i32})  [unwired: 1 in]
            n203 = property class="Pane"(reference=w493, "Origin"=w488) -> (error out=w482:errorcluster)  [unwired: 1 in, 1 out]
            n204 = Close Reference(reference=w487, error in (no error)=w482) -> (error out=w486:errorcluster)
            n205 = Close Reference(reference=w481, error in (no error)=w482) -> (error out=w483:errorcluster)
            n206 = Close Reference(reference=w485, error in (no error)=w486) -> (error out=w478:errorcluster)
            n207 = Close Reference(reference=w480, error in (no error)=w483) -> (error out=w484:errorcluster)
            n208 = Close Reference(reference=w477, error in (no error)=w478) -> (error out=w473:errorcluster)
            n209 = Close Reference(reference=w479, error in (no error)=w484) -> (error out=w474:errorcluster)
            n210 = stacked-sequence {
              tunnel: w474 -> [_]
              tunnel: w473 -> [_]
              frame #0 {
              }
            }
          }
          frame "SaveVI" {
            n211 = Unbundle By Name(w540) -> ("ViRef"=w539:refnum<vi>)
            n212 = call <resource>:"Scripting_SaveVi.vi"("error in (no error)"=w538, "VIRefToSaveIn"=w539) -> ("error out"=w537:errorcluster)  [unwired: 8 in, 1 out]
          }
          frame "CloseReferences", "Error" {
            n213 = call <resource>:"GDSError_LogErrorInformation.vi"("State"=w542, "LocalVariableData"=w543, "error in (no error)"=w544) -> ()  [unwired: 16 in, 1 out]
            n214 = property class="VI"(reference=w552) -> ("Name"=w551:string)  [unwired: 1 in, 2 out]
            n215 = Variant To Data(type=path "", Variant=w554) -> (data=w550:path, error out=w553:errorcluster)  [unwired: 1 in]
            n216 = Strip Path(path=w550) -> (name=w549:string)  [unwired: 1 out]
            n217 = Unbundle By Name(w543) -> ("TemplateClass"=w545:refnum<vi>)
            n218 = disable-structure shown="Enabled" {
              disable-tunnel: w551 -> [w560 _]
              disable-tunnel: w549 -> [w559 _]
              disable-tunnel: w544 -> [w558 _]
              disable-tunnel: w542 -> [w557 _]
              frame Disabled {
                n219 = case shown="Error" w558 {
                  selector: w558 -> [_ w565]
                  tunnel: w559 -> [_ w567]
                  tunnel: w557 -> [_ w563]
                  tunnel: w560 -> [_ w566]
                  frame No Error {
                    n220 = stacked-sequence {
                      frame #0 {
                        n221 = Wait (ms)(milliseconds to wait=u32 2) -> ()  [unwired: 1 out]
                      }
                    }
                  }
                  frame Error {
                    w571 = path "c:/GDS_Error.txt" ("file (use dialog)")
                    n222 = Unbundle(w565) -> ("code"=w562:i32, "source"=w564:string)  [unwired: 1 out]
                    n223 = Read from Text File(file (use dialog)=w571) -> (text=w568:string)  [unwired: 3 in, 3 out]
                    n224 = Format Into String(format string="       %s(%s)Code:%d:%s:%s\n", initial string=w568, w567, w566, w562, w563, w564) -> (resulting string=w570:string)  [unwired: 1 in, 1 out]
                    n225 = stacked-sequence {
                      tunnel: w570 -> [w574]
                      tunnel: w571 -> [w572]
                      frame #0 {
                        n226 = Delete(path (use dialog)=w572) -> (deleted path=w573:path)  [unwired: 4 in, 2 out]
                        n227 = Write to Text File(file (use dialog)=w573, text=w574) -> ()  [unwired: 2 in, 3 out]
                      }
                    }
                    n228 = call <vilib>:"Beep.vi"() -> ()  [unwired: 12 in]
                  }
                }
              }
              frame Enabled {
              }
            }
            n229 = Close Reference(reference=w545) -> (error out=w546:errorcluster)  [unwired: 1 in]
            n230 = case shown="No Error" w553 {
              tunnel: w543 -> [w581 _]
              tunnel: w544 -> [w579 w582]
              tunnel: [w578 w582] -> w548
              tunnel: w546 -> [_ _]
              frame No Error {
                n231 = Unbundle By Name(w581) -> ("TemplateRef"=w580:refnum<vi>)
                n232 = Close Reference(reference=w580, error in (no error)=w579) -> (error out=w578:errorcluster)
              }
              frame Error {
              }
            }
            n233 = stacked-sequence {
              tunnel: w543 -> [w577]
              tunnel: w548 -> [w575]
              tunnel: [w575] -> w547
              frame #0 {
                n234 = Unbundle By Name(w577) -> ("Class"=w576:refnum<vi>)
                n235 = call <resource>:"GDSLvClass_SaveEverythingInClass.vi"("ClassRefIn"=w576) -> ()  [unwired: 17 in, 2 out]
              }
            }
          }
        }
        n236 = Equal?(x=w28, y="Exit") -> (x = y?=w31:bool)
        n237 = Select(t="Error", s=w20, f=w28) -> (s? t:f=w32:string)
      }
    }
    frame Error {
    }
  }
  "error out" <- w10
  n238 = Unbundle By Name(w6) -> ("permissions"=w2:i16, "TemplateFile"=w4:path, "TemplateVersionUsed"=→"TemplateVersionUsed":string)
  n239 = Empty String/Path?(string/path=w4) -> (empty?=w5:bool)
  n240 = case shown="False" w5 {
    tunnel: w4 -> [w585 _]
    tunnel: w2 -> [w584 _]
    frame False {
      n241 = Set Permissions(7:w584, 11:w585) -> ()  [unwired: 3 in, 2 out]
    }
    frame True {
    }
  }
